vi "IMAQ FPGA Camera Link Line Builder (4 Tap U16 4X-1Y).vi"(8 "Input Valid In":bool=TRUE, 9 "Frame Valid In":bool, 10 "Line Valid In":bool, 11 "Pixel Data In":u16[](array[numeric])=[0, 0, 0, 0]) -> (0 "Output Valid":bool, 1 "Frame Valid Out":bool, 2 "Line Valid Out":bool, 3 "Pixel Bus x8 Out":cluster{"Pixels":u16[], "DV":bool[]}, 5 "Overflow":bool)   [LabVIEW 2020]
doc: "Camera Link cameras may return pixels from different parts of the image on each pixel clock. The Line Builder takes those pixels and combines them over multiple cycles to return a Pixel Bus of 8 pixels that are adjacent to each other. \n\nThis instance expects a camera with 4 taps (i.e. 4 pixels returned on each pixel clock). The first tap represents the left quarter of the image and the first valid pixel from this tap is located on the left of the image (pixels 0). The next tap represents the next quarter of the image and the first valid pixel from this tap is located at Width/4 of the image. The next tap represents the next quarter of the image and the first valid pixels from this tap is located in the middle of the image (width/2). The last tap represent the last quarter of the image and the first valid pixel from this tap is located at 3/4*Width of the image."
uses:
  <vilib>/visionFPGA/Basics/Camera Link Acquisition/Controls/IMAQ FPGA Camera Link Line Builder State.ctl
  <vilib>/rvi/Emulation/niFpgaSctlEmulationGetInTimedLoop.vi
  <vilib>/Utility/error.llb/Clear Errors.vi
  <vilib>/rvi/DataTransferAndStorage/Container/Common/niFpgaContainerGetUniqueNameForEmu.vi
  <vilib>/rvi/DataTransferAndStorage/Container/Common/niFpgaContainerSetEmuInfo.vi
  <vilib>/rvi/eio/common/nirviEmuReportErrorAndStop.vi
  <vilib>/rvi/DataTransferAndStorage/Container/Common/niFpgaContainerExecOnDevCompGetState.vi
  <vilib>/rvi/Emulation/niFpgaEmulationIsFPGAContextNoSignature.vi
  <vilib>/rvi/Emulation/niFpgaProcessEmulError.vi
  <vilib>/rvi/errors/nirviReportUnexpectedCaseInternalError (U32).vi
  <vilib>/rvi/Memory/Memory_Emulation/niFpgaMemoryEmulationCacheClearOnFirstRun.vi
  <vilib>/rvi/Memory/Memory_Emulation/nirvimemoryEmulationManagerCache_MakeExclusive.vi
  <vilib>/rvi/Memory/Memory_Emulation/niFpgaMemoryEmulationValidateCache.vi
  <vilib>/rvi/Memory/Memory_Emulation/nirvimemoryEmulationManagerCache_InsertValue.vi
  <vilib>/rvi/Memory/Memory_Emulation/nirvimemoryEmulationManagerCache_ReleaseExclusive.vi
  <vilib>/rvi/Memory/Memory_Emulation/nirvimemoryEmulationManagerCache_GetValue.vi
  <vilib>/rvi/Memory/Memory_Emulation/nirvimemoryEmulationManagerCache_SetValue.vi
  <vilib>/rvi/Emulation/niFpgaSctlEmulationResourceMgr.vi
  <vilib>/rvi/LocalResourceManager/LocalResourceManager.xnode
  <vilib>/rvi/DataTransferAndStorage/Container/XNode/niFpgaContainer.xnode
  <vilib>/rvi/Memory/Memory_Emulation/niFpgaMemoryEmulationRefIn.vi
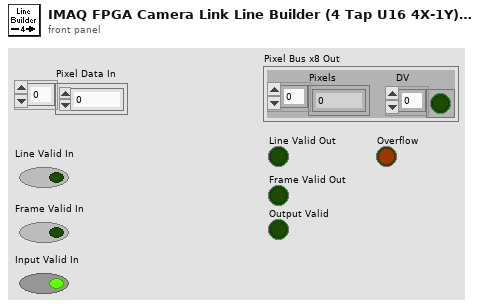
[diagram p1: front panel]
types:
  T1 = typedef "IMAQ FPGA Camera Link Line Builder State.ctl" = enum16{"Wait for First Valid Pixels", "Update Section 1", "Update Section 2", "Update Section 3", "Update Last Section", "Add Final Pack", "Add End of Line", "Check End of Image"}
  T2 = cluster{bool, u16, "Falling Edge":bool, bool, "Falling Edge":bool}
  T3 = cluster{bool, u16, "Falling Edge":bool, "Enum":T1, "Falling Edge":bool}
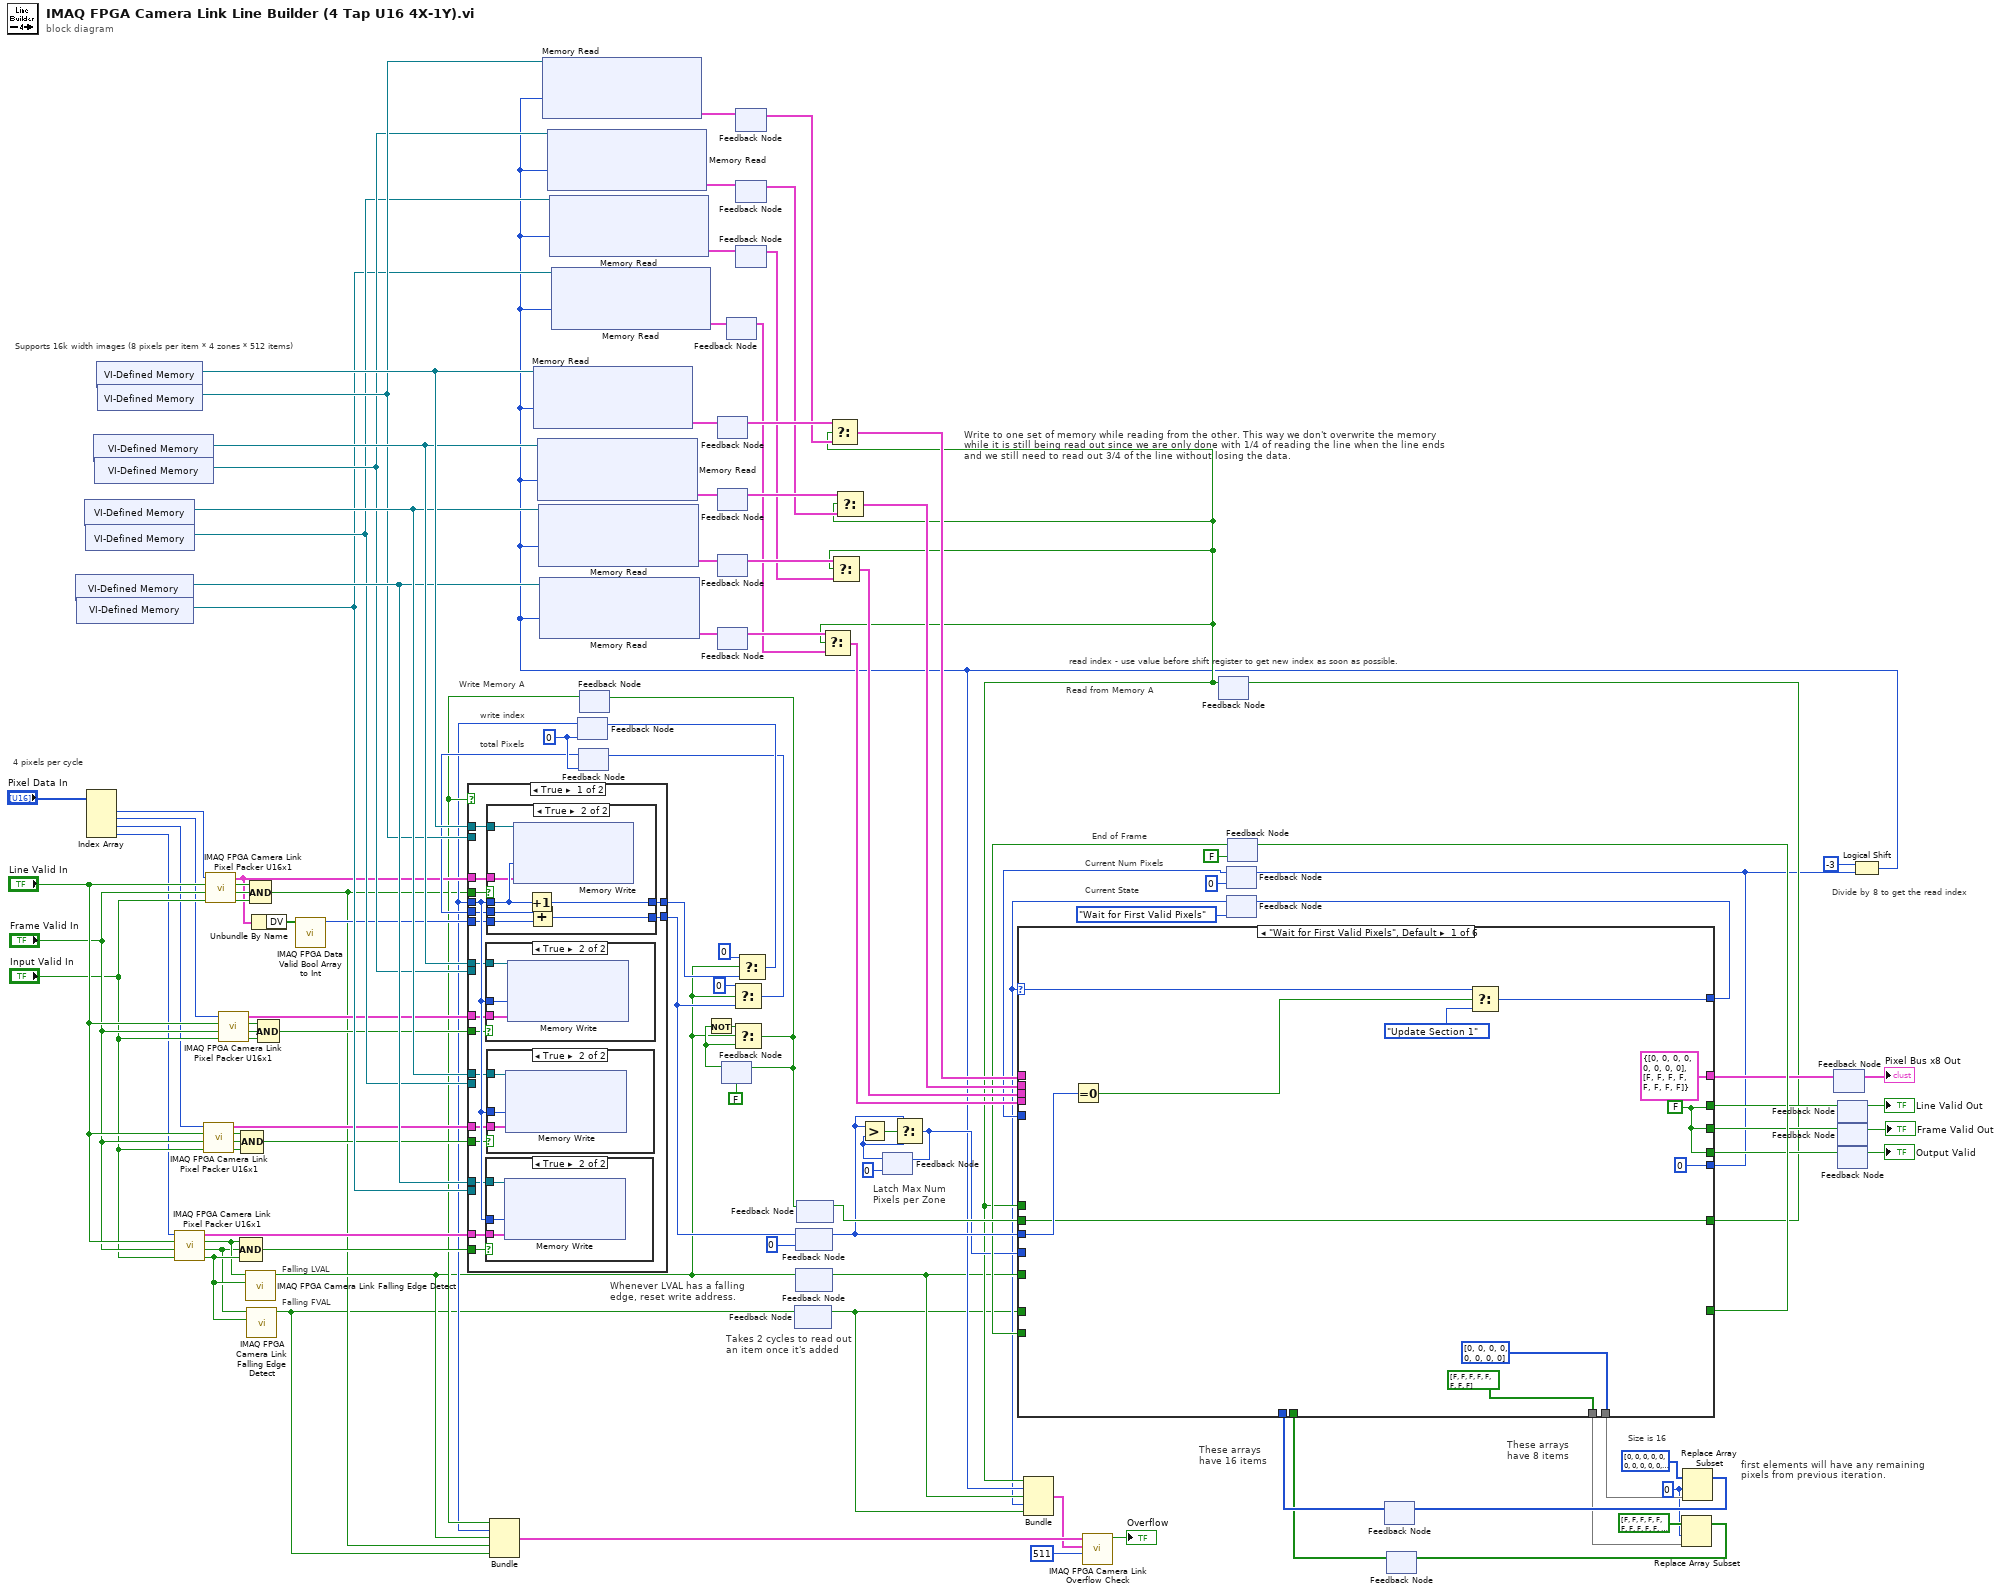
[diagram p0: block diagram]
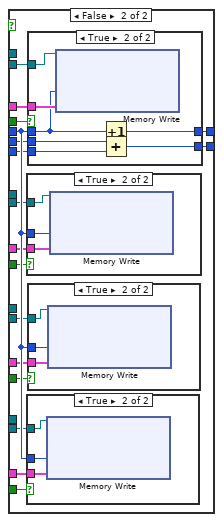
[diagram p6: hidden frame]
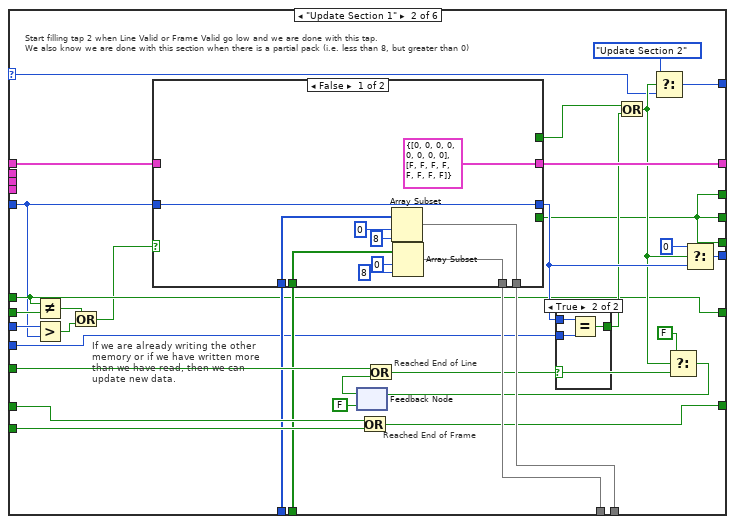
[diagram p11: hidden frame]
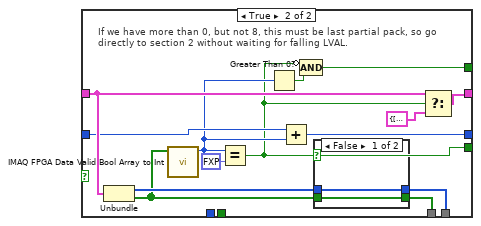
[diagram p12: hidden frame]
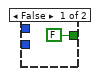
[diagram p14: hidden frame]
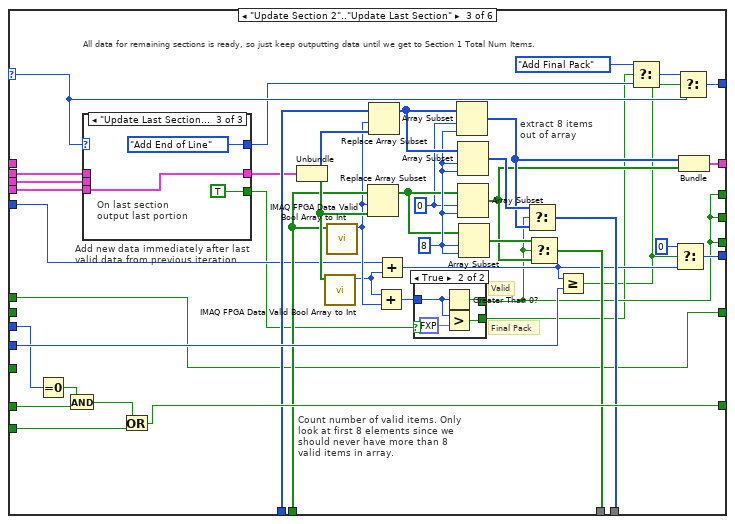
[diagram p15: hidden frame]
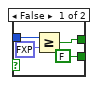
[diagram p16: hidden frame]
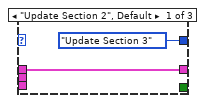
[diagram p17: hidden frame]
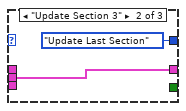
[diagram p18: hidden frame]
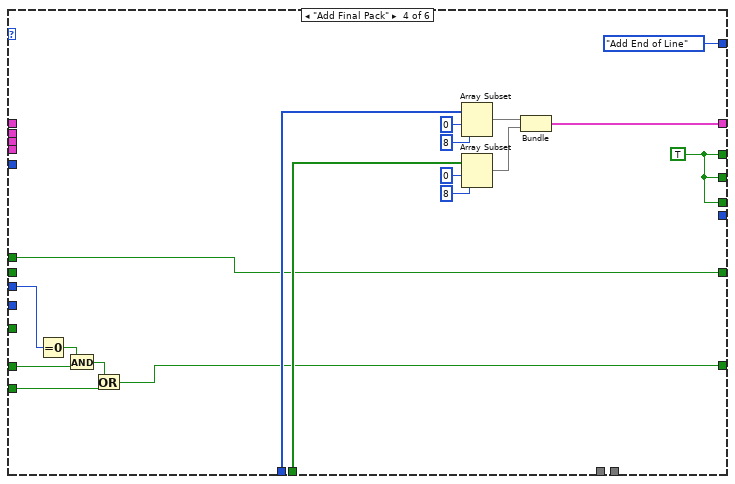
[diagram p19: hidden frame]
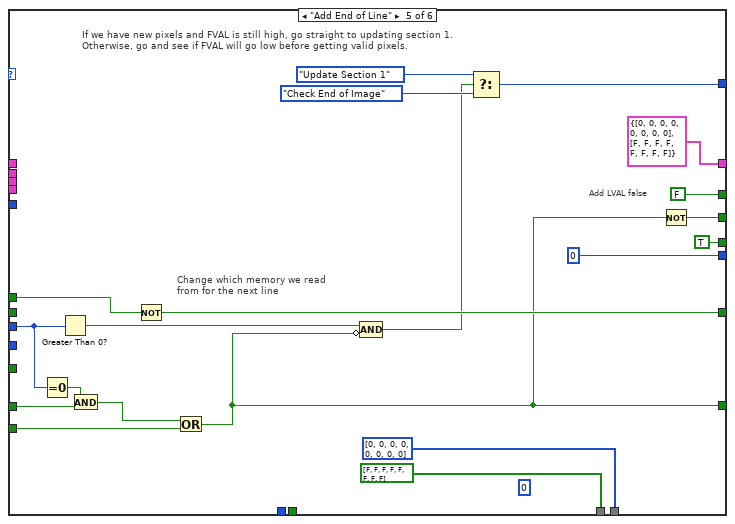
[diagram p20: hidden frame]
diagram:
  w45 = 0 ("index")
  w41 = u16 0
  # "Divide by 8 to get the read index"
  # "Latch Max Num Pixels per Zone"
  # "total Pixels"
  # "These arrays have 8 items"
  # "These arrays have 16 items"
  # "first elements will have any remaining pixels from previous iteration."
  # "Size is 16"
  # "Read from Memory A"
  # "Write Memory A"
  # "Write to one set of memory while reading from the other. This way we don't overwrite the memory while it is still being read out since we are only done with 1/4 of reading the line when the line ends and we still need to read out 3/4 of the line without losing the data."
  # "Falling FVAL"
  # "Falling LVAL"
  # "read index - use value before shift register to get new index as soon as possible."
  # "write index"
  # "Current State"
  # "End of Frame"
  # "Takes 2 cycles to read out an item once it's added"
  # "Current Num Pixels"
  # "Whenever LVAL has a falling edge, reset write address."
  # "Supports 16k width images (8 pixels per item * 4 zones * 512 items)"
  # "4 pixels per cycle"
  n1 = xnode "VI-Defined Memory"() -> ("Memory Out"=w92:refnum<k21>)
  n2 = xnode "VI-Defined Memory"() -> ("Memory Out"=w84:refnum<k21>)
  n3 = xnode "VI-Defined Memory"() -> ("Memory Out"=w93:refnum<k21>)
  n4 = xnode "VI-Defined Memory"() -> ("Memory Out"=w85:refnum<k21>)
  n5 = Index Array(array="Pixel Data In") -> (element #1=w4:u16, element #2=w3:u16, element #3=w2:u16, element #4=w1:u16)  [unwired: 4 in]
  n6 = xnode "VI-Defined Memory"() -> ("Memory Out"=w94:refnum<k21>)
  n7 = xnode "VI-Defined Memory"() -> ("Memory Out"=w86:refnum<k21>)
  n8 = xnode "VI-Defined Memory"() -> ("Memory Out"=w95:refnum<k21>)
  n9 = xnode "VI-Defined Memory"() -> ("Memory Out"=w87:refnum<k21>)
  n10 = call <vilib>:"IMAQ FPGA Camera Link Pixel Packer U16x1.vi"("Input Valid"="Input Valid In", "Frame Valid In"="Frame Valid In", "Line Valid In"="Line Valid In", "Pixel In"=w1) -> ("Output Valid"=w34:bool, "Frame Valid Out"=w32:bool, "Line Valid Out"=w33:bool, "Pixel Bus x8 Out"=w69:cluster{"Pixels":u16[], "DV":bool[]})  [unwired: 4 in]
  n11 = call <vilib>:"IMAQ FPGA Camera Link Pixel Packer U16x1.vi"("Input Valid"="Input Valid In", "Frame Valid In"="Frame Valid In", "Line Valid In"="Line Valid In", "Pixel In"=w2) -> ("Output Valid"=w59:bool, "Frame Valid Out"=w60:bool, "Line Valid Out"=w61:bool, "Pixel Bus x8 Out"=w70:cluster{"Pixels":u16[], "DV":bool[]})  [unwired: 4 in]
  n12 = call <vilib>:"IMAQ FPGA Camera Link Pixel Packer U16x1.vi"("Input Valid"="Input Valid In", "Frame Valid In"="Frame Valid In", "Line Valid In"="Line Valid In", "Pixel In"=w4) -> ("Output Valid"=w109:bool, "Frame Valid Out"=w110:bool, "Line Valid Out"=w111:bool, "Pixel Bus x8 Out"=w35:cluster{"Pixels":u16[], "DV":bool[]})  [unwired: 4 in]
  n13 = call <vilib>:"IMAQ FPGA Camera Link Pixel Packer U16x1.vi"("Input Valid"="Input Valid In", "Frame Valid In"="Frame Valid In", "Line Valid In"="Line Valid In", "Pixel In"=w3) -> ("Output Valid"=w65:bool, "Frame Valid Out"=w64:bool, "Line Valid Out"=w63:bool, "Pixel Bus x8 Out"=w71:cluster{"Pixels":u16[], "DV":bool[]})  [unwired: 4 in]
  n14 = Compound Arithmetic op=AND(w33, w32, w34) -> (w57:bool)
  n15 = Compound Arithmetic op=AND(w61, w60, w59) -> (w58:bool)
  n16 = call <vilib>:"IMAQ FPGA Camera Link Falling Edge Detect.vi"("Input Valid"=w34, "Input"=w33) -> ("Falling Edge"=w16:bool)  [unwired: 9 in]
  n17 = call <vilib>:"IMAQ FPGA Camera Link Falling Edge Detect.vi"("Input Valid"=w34, "Input"=w32) -> ("Falling Edge"=w14:bool)  [unwired: 9 in]
  n18 = Compound Arithmetic op=AND(w111, w110, w109) -> (w15:bool)
  n19 = Unbundle By Name(w35) -> ("DV"=w44:bool[])
  n20 = Compound Arithmetic op=AND(w63, w64, w65) -> (w62:bool)
  n21 = call <vilib>:"IMAQ FPGA Data Valid Bool Array to Int.vi"("DV In"=w44) -> ("Sum DV Out"=w39:u8)  [unwired: 10 in]
  n22 = feedback #1(w41) -> (w17:u16)
  n23 = feedback #2(w41) -> (w40:u16)
  n24 = feedback #3() -> (w18:bool)  [unwired: 1 in]
  n25 = case shown="True" w18 {
    tunnel: [w134 w169] -> w112
    tunnel: w17 -> [w133 w168]
    tunnel: w15 -> [w124 w167]
    tunnel: w35 -> [w132 w166]
    tunnel: w71 -> [w131 w165]
    tunnel: w70 -> [w130 w164]
    tunnel: w69 -> [w129 w163]
    tunnel: w95 -> [w128 _]
    tunnel: w94 -> [w127 _]
    tunnel: w93 -> [w126 _]
    tunnel: w92 -> [w125 _]
    tunnel: w87 -> [_ w162]
    tunnel: w86 -> [_ w161]
    tunnel: w85 -> [_ w160]
    tunnel: w84 -> [_ w159]
    tunnel: w62 -> [w123 w158]
    tunnel: w58 -> [w122 w157]
    tunnel: w57 -> [w121 w156]
    tunnel: [w120 w155] -> w38
    tunnel: w40 -> [w119 w154]
    tunnel: w39 -> [w118 w153]
    frame True {
      n26 = case shown="True" w123 {
        tunnel: w131 -> [_ w142]
        tunnel: w127 -> [_ w143]
        tunnel: w133 -> [_ w141]
        frame False {
        }
        frame True {
          n27 = xnode ("Memory Write")("Address"=w141, "Data"=w142, "Memory In"=w143) -> ()  [unwired: 1 out]
        }
      }
      n28 = case shown="True" w121 {
        tunnel: w129 -> [_ w136]
        tunnel: w125 -> [_ w137]
        tunnel: w133 -> [_ w135]
        frame False {
        }
        frame True {
          n29 = xnode ("Memory Write")("Address"=w135, "Data"=w136, "Memory In"=w137) -> ()  [unwired: 1 out]
        }
      }
      n30 = case shown="True" w124 {
        tunnel: [w144 w146] -> w134
        tunnel: w133 -> [w145 w151]
        tunnel: w128 -> [_ w152]
        tunnel: w132 -> [_ w150]
        tunnel: [w145 w149] -> w120
        tunnel: w119 -> [w144 w148]
        tunnel: w118 -> [_ w147]
        frame False {
        }
        frame True {
          n31 = xnode ("Memory Write")("Address"=w151, "Data"=w150, "Memory In"=w152) -> ()  [unwired: 1 out]
          n32 = Increment(x=w151) -> (x+1=w149:u16)
          n33 = Add(x=w148, y=w147) -> (x+y=w146:u16)
        }
      }
      n34 = case shown="True" w122 {
        tunnel: w130 -> [_ w139]
        tunnel: w126 -> [_ w140]
        tunnel: w133 -> [_ w138]
        frame False {
        }
        frame True {
          n35 = xnode ("Memory Write")("Address"=w138, "Data"=w139, "Memory In"=w140) -> ()  [unwired: 1 out]
        }
      }
    }
    frame False {
      n36 = case shown="True" w158 {
        tunnel: w165 -> [_ w177]
        tunnel: w161 -> [_ w178]
        tunnel: w168 -> [_ w176]
        frame False {
        }
        frame True {
          n37 = xnode ("Memory Write")("Address"=w176, "Data"=w177, "Memory In"=w178) -> ()  [unwired: 1 out]
        }
      }
      n38 = case shown="True" w156 {
        tunnel: w163 -> [_ w171]
        tunnel: w159 -> [_ w172]
        tunnel: w168 -> [_ w170]
        frame False {
        }
        frame True {
          n39 = xnode ("Memory Write")("Address"=w170, "Data"=w171, "Memory In"=w172) -> ()  [unwired: 1 out]
        }
      }
      n40 = case shown="True" w167 {
        tunnel: [w179 w183] -> w169
        tunnel: w168 -> [w180 w185]
        tunnel: w162 -> [_ w187]
        tunnel: w166 -> [_ w186]
        tunnel: [w180 w184] -> w155
        tunnel: w154 -> [w179 w182]
        tunnel: w153 -> [_ w181]
        frame False {
        }
        frame True {
          n41 = xnode ("Memory Write")("Address"=w185, "Data"=w186, "Memory In"=w187) -> ()  [unwired: 1 out]
          n42 = Increment(x=w185) -> (x+1=w184:u16)
          n43 = Add(x=w182, y=w181) -> (x+y=w183:u16)
        }
      }
      n44 = case shown="True" w157 {
        tunnel: w164 -> [_ w174]
        tunnel: w160 -> [_ w175]
        tunnel: w168 -> [_ w173]
        frame False {
        }
        frame True {
          n45 = xnode ("Memory Write")("Address"=w173, "Data"=w174, "Memory In"=w175) -> ()  [unwired: 1 out]
        }
      }
    }
  }
  n46 = Bundle(w18, w17, "Falling Edge"=w16, w15, "Falling Edge"=w14) -> (w13:T2)  [unwired: 1 in]
  n47 = feedback #4() -> (w79:cluster{"Pixels":u16[], "DV":bool[]})  [unwired: 1 in]
  n48 = feedback #5() -> (w77:cluster{"Pixels":u16[], "DV":bool[]})  [unwired: 1 in]
  n49 = feedback #6() -> (w75:cluster{"Pixels":u16[], "DV":bool[]})  [unwired: 1 in]
  n50 = feedback #7() -> (w73:cluster{"Pixels":u16[], "DV":bool[]})  [unwired: 1 in]
  n51 = feedback #8(FALSE) -> (w43:bool)
  n52 = Not(x=w43) -> (.not. x?=w107:bool)
  n53 = feedback #9() -> (w72:cluster{"Pixels":u16[], "DV":bool[]})  [unwired: 1 in]
  n54 = Select(t=u16 0, s=w16, f=w112) -> (s? t:f=w36:u16)
  n55 = feedback-in #2(w36) -> ()
  n56 = Select(t=w107, s=w16, f=w43) -> (s? t:f=w31:bool)
  n57 = feedback-in #3(w31) -> ()
  n58 = feedback-in #8(w31) -> ()
  n59 = feedback #10() -> (w78:cluster{"Pixels":u16[], "DV":bool[]})  [unwired: 1 in]
  n60 = feedback #11() -> (w76:cluster{"Pixels":u16[], "DV":bool[]})  [unwired: 1 in]
  n61 = feedback #12() -> (w74:cluster{"Pixels":u16[], "DV":bool[]})  [unwired: 1 in]
  n62 = Select(t=u16 0, s=w16, f=w38) -> (s? t:f=w37:u16)
  n63 = feedback-in #1(w37) -> ()
  n64 = feedback #13() -> (w7:bool)  [unwired: 1 in]
  n65 = feedback-in #13(w14) -> ()
  n66 = feedback-in #14(w112) -> ()
  n67 = feedback #14(u16 0) -> (w29:u16)
  n68 = feedback-in #15(w16) -> ()
  n69 = feedback #15() -> (w10:bool)  [unwired: 1 in]
  n70 = feedback #16() -> (w49:bool)  [unwired: 1 in]
  n71 = feedback-in #16(w31) -> ()
  n72 = feedback #17(u16 0) -> (w28:u16)
  n73 = Greater?(x=w29, y=w28) -> (0:w30:bool)
  n74 = Select(t=w29, s=w30, f=w28) -> (s? t:f=w19:u16)
  n75 = feedback-in #17(w19) -> ()
  n76 = feedback #18() -> (w12:bool)  [unwired: 1 in]
  n77 = Select(t=w73, s=w12, f=w72) -> (s? t:f=w66:cluster{"Pixels":u16[], "DV":bool[]})
  n78 = Select(t=w79, s=w12, f=w78) -> (s? t:f=w48:cluster{"Pixels":u16[], "DV":bool[]})
  n79 = Select(t=w75, s=w12, f=w74) -> (s? t:f=w67:cluster{"Pixels":u16[], "DV":bool[]})
  n80 = Select(t=w77, s=w12, f=w76) -> (s? t:f=w68:cluster{"Pixels":u16[], "DV":bool[]})
  n81 = feedback #19(u16 0) -> (w21:u16)
  n82 = feedback #20(IMAQ_FPGA_Camera_Link_Line_Builder_State."Wait for First Valid Pixels" ("Enum")) -> (w8:T1)
  n83 = feedback #21(FALSE) -> (w23:bool)
  n84 = feedback #22() -> (w47:u16[])  [unwired: 1 in]
  n85 = feedback #23() -> (w46:bool[])  [unwired: 1 in]
  n86 = case shown="\"Wait for First Valid Pixels\", Default" w8 {
    selector: w8 -> [w198 w199 w290 _ _ w377]
    tunnel: [w197 w231 w304 IMAQ_FPGA_Camera_Link_Line_Builder_State."Add End of Line" ("Enum") w352 w378] -> w20
    tunnel: w10 -> [_ w229 _ _ _ _]
    tunnel: w7 -> [_ w225 w270 w321 w341 w364]
    tunnel: [u16 0 w228 w300 _ u16 0 u16 0] -> w26
    tunnel: w21 -> [_ w205 w277 _ _ _]
    tunnel: w29 -> [w193 w206 w271 w322 w342 w365]
    tunnel: w19 -> [_ w218 w301 _ _ _]
    tunnel: [_ w221 w302 w324 w338 w374] -> w113
    tunnel: w23 -> [_ w226 w303 w325 w356 w380]
    tunnel: w48 -> [_ w215 _ _ _ _]
    tunnel: w68 -> [_ _ w292 _ _ _]
    tunnel: w67 -> [_ _ w289 _ _ _]
    tunnel: w66 -> [_ _ w288 _ _ _]
    tunnel: w49 -> [w192 w208 _ _ _ w361]
    tunnel: [w192 w209 w264 w326 w347 w360] -> w50
    tunnel: w12 -> [_ w209 w264 w326 w348 w360]
    tunnel: w46 -> [_ w219 w287 w329 _ _]
    tunnel: w47 -> [_ w220 w296 w330 _ _]
    tunnel: [cluster{"Pixels":u16[], "DV":bool[]} {"Pixels"=[0, 0, 0, 0, 0, 0, 0, 0], "DV"=[FALSE, FALSE, FALSE, FALSE, FALSE, FALSE, FALSE, FALSE]} ("Data") w224 w299 w328 cluster{"Pixels":u16[], "DV":bool[]} {"Pixels"=[0, 0, 0, 0, 0, 0, 0, 0], "DV"=[FALSE, FALSE, FALSE, FALSE, FALSE, FALSE, FALSE, FALSE]} ("Data") cluster{"Pixels":u16[], "DV":bool[]} {"Pixels"=[0, 0, 0, 0, 0, 0, 0, 0], "DV"=[FALSE, FALSE, FALSE, FALSE, FALSE, FALSE, FALSE, FALSE]} ("Data")] -> w103
    tunnel: [w188 w202 w267 w327 FALSE FALSE] -> w101
    tunnel: [w188 w202 w267 w327 w349 w370] -> w100
    tunnel: [w188 w202 w267 w327 TRUE TRUE] -> w99
    tunnel: [bool[] [FALSE, FALSE, FALSE, FALSE, FALSE, FALSE, FALSE, FALSE] ("DV") w223 w281 _ bool[] [FALSE, FALSE, FALSE, FALSE, FALSE, FALSE, FALSE, FALSE] bool[] [FALSE, FALSE, FALSE, FALSE, FALSE, FALSE, FALSE, FALSE]] -> w51
    tunnel: [u16[] [0, 0, 0, 0, 0, 0, 0, 0] ("Pixels") w222 w280 _ u16[] [0, 0, 0, 0, 0, 0, 0, 0] ("Pixels") u16[] [0, 0, 0, 0, 0, 0, 0, 0] ("Pixels")] -> w52
    frame "Wait for First Valid Pixels", Default {
      w188 = FALSE
      n87 = Equal To 0?(x=w193) -> (x = 0?=w196:bool)
      n88 = Select(t=w198, s=w196, f=IMAQ_FPGA_Camera_Link_Line_Builder_State."Update Section 1") -> (s? t:f=w197:T1)
    }
    frame "Update Section 1" {
      # "If we are already writing the other memory or if we have written more than we have read, then we can update new data."
      # "Reached End of Frame"
      # "Reached End of Line"
      # "Start filling tap 2 when Line Valid or Frame Valid go low and we are done with this tap.\nWe also know we are done with this section when there is a partial pack (i.e. less than 8, but greater than 0)"
      n89 = Not Equal?(x=w209, y=w208) -> (x != y?=w207:bool)
      n90 = Greater?(x=w206, y=w205) -> (0:w204:bool)
      n91 = Or(x=w207, y=w204) -> (x .or. y?=w203:bool)
      n92 = case shown="False" w203 {
        tunnel: w215 -> [_ w252]
        tunnel: w205 -> [w241 w250]
        tunnel: [w241 w255] -> w227
        tunnel: [cluster{"Pixels":u16[], bool[]} {"Pixels"=[0, 0, 0, 0, 0, 0, 0, 0], [FALSE, FALSE, FALSE, FALSE, FALSE, FALSE, FALSE, FALSE]} w254] -> w224
        tunnel: [w232 w245] -> w223
        tunnel: [w236 w246] -> w222
        tunnel: w220 -> [w239 _]
        tunnel: w219 -> [w235 _]
        tunnel: [_ w244] -> w202
        tunnel: [_ w242] -> w201
        frame False {
          n93 = Array Subset(array=w239, index=0, length=8) -> (w236:u16[])
          n94 = Array Subset(array=w235, index=0, length=8) -> (w232:bool[])
        }
        frame True {
          # "If we have more than 0, but not 8, this must be last partial pack, so go directly to section 2 without waiting for falling LVAL."
          n95 = Unbundle(w252) -> ("Pixels"=w248:u16[], "DV"=w247:bool[])
          n96 = call <vilib>:"IMAQ FPGA Data Valid Bool Array to Int.vi"("DV In"=w247) -> ("Sum DV Out"=w249:u8)  [unwired: 10 in]
          n97 = Equal?(x=w249, y=fxp<+,4,4> 8.0) -> (x = y?=w244:bool)
          n98 = Greater Than 0?(x=w249) -> (x > 0?=w243:bool)
          n99 = Add(x=w250, y=w249) -> (x+y=w255:u16)
          n100 = Compound Arithmetic op=AND(invert w244, w243) -> (w242:bool)
          n101 = case shown="False" w244 {
            tunnel: w248 -> [w257 _]
            tunnel: w247 -> [w256 _]
            tunnel: [w257 _] -> w246
            tunnel: [w256 _] -> w245
            frame False {
            }
            frame True {
            }
          }
          n102 = Select(t=w252, s=w244, f=cluster{"Pixels":u16[], "DV":bool[]} {"Pixels"=[0, 0, 0, 0, 0, 0, 0, 0], "DV"=[FALSE, FALSE, FALSE, FALSE, FALSE, FALSE, FALSE, FALSE]}) -> (s? t:f=w254:cluster{"Pixels":u16[], "DV":bool[]})
        }
      }
      n103 = feedback #24(FALSE) -> (w214:bool)
      n104 = Or(x=w225, y=w226) -> (x .or. y?=w221:bool)
      n105 = Or(x=w229, y=w214) -> (x .or. y?=w213:bool)
      n106 = case shown="True" w213 {
        tunnel: w218 -> [_ w260]
        tunnel: w227 -> [_ w261]
        tunnel: [FALSE w259] -> w216
        frame False {
        }
        frame True {
          n107 = Equal?(x=w261, y=w260) -> (x = y?=w259:bool)
        }
      }
      n108 = Or(x=w201, y=w216) -> (x .or. y?=w212:bool)
      n109 = Select(t=IMAQ_FPGA_Camera_Link_Line_Builder_State."Update Section 2" ("Enum"), s=w212, f=w199) -> (s? t:f=w231:T1)
      n110 = Select(t=FALSE, s=w212, f=w213) -> (s? t:f=w210:bool)
      n111 = feedback-in #24(w210) -> ()
      n112 = Select(t=u16 0, s=w212, f=w227) -> (s? t:f=w228:u16)
    }
    frame "Update Section 2".."Update Last Section" {
      w279 = 0 ("index")
      w294 = 8 ("length")
      # "Final Pack"
      # "Valid"
      # "extract 8 items out of array"
      # "Add new data immediately after last valid data from previous iteration."
      # "Count number of valid items. Only look at first 8 elements since we should never have more than 8 valid items in array."
      # "All data for remaining sections is ready, so just keep outputting data until we get to Section 1 Total Num Items."
      n113 = Equal To 0?(x=w271) -> (x = 0?=w272:bool)
      n114 = And(x=w272, y=w270) -> (x .and. y?=w269:bool)
      n115 = case shown="\"Update Last Section\"" w290 {
        tunnel: w292 -> [w314 _ _]
        tunnel: [w314 w315 w318] -> w291
        tunnel: [IMAQ_FPGA_Camera_Link_Line_Builder_State."Update Section 3" ("t") IMAQ_FPGA_Camera_Link_Line_Builder_State."Update Last Section" ("t") IMAQ_FPGA_Camera_Link_Line_Builder_State."Add End of Line" ("t")] -> w275
        tunnel: w289 -> [_ w315 _]
        tunnel: w288 -> [_ _ w318]
        tunnel: [_ _ TRUE] -> w268
        frame "Update Section 2", Default {
        }
        frame "Update Section 3" {
        }
        frame "Update Last Section" {
          # "On last section output last portion"
        }
      }
      n116 = Or(x=w269, y=w303) -> (x .or. y?=w302:bool)
      n117 = Unbundle(w291) -> ("Pixels"=w298:u16[], "DV"=w297:bool[])
      n118 = call <vilib>:"IMAQ FPGA Data Valid Bool Array to Int.vi"("DV In"=w297) -> ("Sum DV Out"=w276:u8)  [unwired: 10 in]
      n119 = call <vilib>:"IMAQ FPGA Data Valid Bool Array to Int.vi"("DV In"=w287) -> ("Sum DV Out"=w286:u8)  [unwired: 10 in]
      n120 = Replace Array Subset(array=w287, new element=w297, index=w286) -> (w293:bool[])
      n121 = Replace Array Subset(array=w296, new element=w298, index=w286) -> (w295:u16[])
      n122 = Add(x=w276, y=w286) -> (x+y=w265:u8)
      n123 = Add(x=w277, y=w276) -> (x+y=w278:u16)
      n124 = case shown="True" w268 {
        tunnel: [w308 w312] -> w267
        tunnel: [FALSE w310] -> w266
        tunnel: w265 -> [w305 w309]
        frame False {
          n125 = Greater Or Equal?(x=w305, y=fxp<+,5,5> 8.0) -> (x >= y?=w308:bool)
        }
        frame True {
          n126 = Greater Than 0?(x=w309) -> (x > 0?=w312:bool)
          n127 = Greater?(x=w309, y=fxp<+,5,5> 8.0) -> (0:w310:bool)
        }
      }
      n128 = Array Subset(array=w295, index=w279, length=w294) -> (w284:u16[])
      n129 = Array Subset(array=w295, index=w294, length=w294) -> (w285:u16[])
      n130 = Array Subset(array=w293, index=w279, length=w294) -> (w282:bool[])
      n131 = Array Subset(array=w293, index=w294, length=w294) -> (w283:bool[])
      n132 = Select(t=w285, s=w267, f=w284) -> (s? t:f=w280:u16[])
      n133 = Select(t=w283, s=w267, f=w282) -> (s? t:f=w281:bool[])
      n134 = Greater Or Equal?(x=w278, y=w301) -> (x >= y?=w263:bool)
      n135 = Select(t=IMAQ_FPGA_Camera_Link_Line_Builder_State."Add Final Pack", s=w266, f=w275) -> (s? t:f=w274:T1)
      n136 = Select(t=u16 0, s=w263, f=w278) -> (s? t:f=w300:u16)
      n137 = Select(t=w274, s=w263, f=w290) -> (s? t:f=w304:T1)
      n138 = Bundle(w284, w282) -> (w299:cluster{u16[], bool[]})  [unwired: 1 in]
    }
    frame "Add Final Pack" {
      w327 = TRUE
      n139 = Equal To 0?(x=w322) -> (x = 0?=w323:bool)
      n140 = And(x=w323, y=w321) -> (x .and. y?=w320:bool)
      n141 = Or(x=w320, y=w325) -> (x .or. y?=w324:bool)
      n142 = Array Subset(array=w330, index=0, length=8) -> (w332:u16[])
      n143 = Array Subset(array=w329, index=0, length=8) -> (w331:bool[])
      n144 = Bundle(w332, w331) -> (w328:cluster{u16[], bool[]})  [unwired: 1 in]
    }
    frame "Add End of Line" {
      (unwired) i8 0
      # "Change which memory we read from for the next line"
      # "Add LVAL false"
      # "If we have new pixels and FVAL is still high, go straight to updating section 1. Otherwise, go and see if FVAL will go low before getting valid pixels."
      n145 = Equal To 0?(x=w342) -> (x = 0?=w343:bool)
      n146 = Greater Than 0?(x=w342) -> (x > 0?=w355:bool)
      n147 = And(x=w343, y=w341) -> (x .and. y?=w340:bool)
      n148 = Not(x=w348) -> (.not. x?=w347:bool)
      n149 = Or(x=w340, y=w356) -> (x .or. y?=w338:bool)
      n150 = Compound Arithmetic op=AND(w355, invert w338) -> (w339:bool)
      n151 = Select(t=IMAQ_FPGA_Camera_Link_Line_Builder_State."Update Section 1" ("Enum"), s=w339, f=IMAQ_FPGA_Camera_Link_Line_Builder_State."Check End of Image" ("Enum")) -> (s? t:f=w352:T1)
      n152 = Not(x=w338) -> (.not. x?=w349:bool)
    }
    frame "Check End of Image" {
      # "If not reading from same memory or there's already data, go straight to Updating Section 1."
      # "Stay in this state until we get new pixels, or we get end of image"
      # "End of Image"
      n153 = Equal To 0?(x=w365) -> (x = 0?=w366:bool)
      n154 = Greater Than 0?(x=w365) -> (x > 0?=w362:bool)
      n155 = Not Equal?(x=w360, y=w361) -> (x != y?=w359:bool)
      n156 = And(x=w366, y=w364) -> (x .and. y?=w363:bool)
      n157 = Or(x=w359, y=w362) -> (x .or. y?=w358:bool)
      n158 = Or(x=w363, y=w380) -> (x .or. y?=w371:bool)
      n159 = Select(t=IMAQ_FPGA_Camera_Link_Line_Builder_State."Update Section 1" ("Enum"), s=w358, f=IMAQ_FPGA_Camera_Link_Line_Builder_State."Wait for First Valid Pixels" ("Enum")) -> (s? t:f=w379:T1)
      n160 = Or(x=w358, y=w371) -> (x .or. y?=w376:bool)
      n161 = Select(t=w379, s=w376, f=w377) -> (s? t:f=w378:T1)
      n162 = Select(t=FALSE, s=w376, f=w371) -> (s? t:f=w374:bool)
      n163 = Not(x=w371) -> (.not. x?=w370:bool)
    }
  }
  n164 = feedback-in #18(w50) -> ()
  n165 = feedback-in #19(w26) -> ()
  n166 = feedback-in #20(w20) -> ()
  n167 = feedback-in #21(w113) -> ()
  n168 = Replace Array Subset(array=bool[] [FALSE, FALSE, FALSE, FALSE, FALSE, FALSE, FALSE, FALSE, FALSE, FALSE, FALSE, FALSE, FALSE, FALSE, FALSE, FALSE], new element=w51, index=w45) -> (w53:bool[])
  n169 = feedback-in #23(w53) -> ()
  n170 = Replace Array Subset(array=u16[] [0, 0, 0, 0, 0, 0, 0, 0, 0, 0, 0, 0, 0, 0, 0, 0] ("Pixels"), new element=w52, index=w45) -> (w55:u16[])
  n171 = feedback-in #22(w55) -> ()
  n172 = feedback #25() -> (→"Pixel Bus x8 Out":cluster{"Pixels":u16[], "DV":bool[]})  [unwired: 1 in]
  n173 = feedback-in #25(w103) -> ()
  n174 = feedback #26() -> (→"Line Valid Out":bool)  [unwired: 1 in]
  n175 = feedback-in #26(w101) -> ()
  n176 = feedback #27() -> (→"Frame Valid Out":bool)  [unwired: 1 in]
  n177 = feedback-in #27(w100) -> ()
  n178 = feedback #28() -> (→"Output Valid":bool)  [unwired: 1 in]
  n179 = feedback-in #28(w99) -> ()
  n180 = Logical Shift(y=i16 -3, x=w26) -> (x << y=w11:u16)
  n181 = xnode ("Memory Read")("Address"=w11, "Memory In"=w95) -> ("Data"=w91:cluster{"Pixels":u16[], "DV":bool[]})  [unwired: 1 out]
  n182 = xnode ("Memory Read")("Address"=w11, "Memory In"=w94) -> ("Data"=w90:cluster{"Pixels":u16[], "DV":bool[]})  [unwired: 1 out]
  n183 = xnode ("Memory Read")("Address"=w11, "Memory In"=w93) -> ("Data"=w89:cluster{"Pixels":u16[], "DV":bool[]})  [unwired: 1 out]
  n184 = xnode ("Memory Read")("Address"=w11, "Memory In"=w92) -> ("Data"=w88:cluster{"Pixels":u16[], "DV":bool[]})  [unwired: 1 out]
  n185 = xnode ("Memory Read")("Address"=w11, "Memory In"=w87) -> ("Data"=w80:cluster{"Pixels":u16[], "DV":bool[]})  [unwired: 1 out]
  n186 = xnode ("Memory Read")("Address"=w11, "Memory In"=w86) -> ("Data"=w81:cluster{"Pixels":u16[], "DV":bool[]})  [unwired: 1 out]
  n187 = xnode ("Memory Read")("Address"=w11, "Memory In"=w85) -> ("Data"=w82:cluster{"Pixels":u16[], "DV":bool[]})  [unwired: 1 out]
  n188 = xnode ("Memory Read")("Address"=w11, "Memory In"=w84) -> ("Data"=w83:cluster{"Pixels":u16[], "DV":bool[]})  [unwired: 1 out]
  n189 = feedback-in #4(w91) -> ()
  n190 = feedback-in #5(w90) -> ()
  n191 = feedback-in #6(w89) -> ()
  n192 = feedback-in #7(w88) -> ()
  n193 = feedback-in #9(w83) -> ()
  n194 = feedback-in #10(w80) -> ()
  n195 = feedback-in #11(w81) -> ()
  n196 = feedback-in #12(w82) -> ()
  n197 = Bundle(w12, w11, "Falling Edge"=w10, "Enum"=w8, "Falling Edge"=w7) -> (w9:T3)  [unwired: 1 in]
  n198 = call <vilib>:"IMAQ FPGA Camera Link Overflow Check.vi"("Max Index"=u16 511, "Read Info"=w9, "Write Info"=w13) -> ("Overlfow"=→"Overflow":bool)  [unwired: 8 in]
